vi "ShoulderNetwork.vi"(8 "error in (no error)":errorcluster) -> (0 "error out":errorcluster)   [LabVIEW 2023]
uses:
  Elevator/ElevatorGlobal.vi
  <vilib>/Rock Robotics/Network Tables/NT Write Boolean.vi
  <vilib>/Rock Robotics/Network Tables/NT Write Number.vi
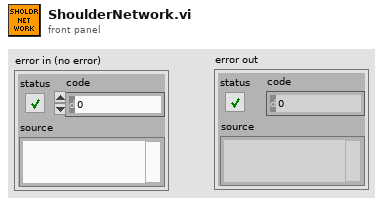
[diagram p1: front panel]
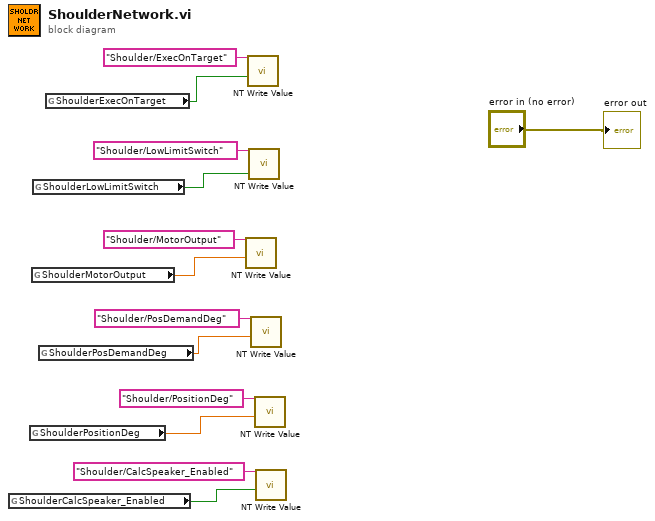
[diagram p0: block diagram]
diagram:
  n1 = global read "ElevatorGlobal.vi" "ShoulderCalcSpeaker_Enabled"() -> (w9:bool)
  n2 = global read "ElevatorGlobal.vi" "ShoulderPositionDeg"() -> (w5:dbl)
  n3 = global read "ElevatorGlobal.vi" "ShoulderMotorOutput"() -> (w3:dbl)
  n4 = global read "ElevatorGlobal.vi" "ShoulderLowLimitSwitch"() -> (w2:bool)
  n5 = global read "ElevatorGlobal.vi" "ShoulderPosDemandDeg"() -> (w4:dbl)
  n6 = global read "ElevatorGlobal.vi" "ShoulderExecOnTarget"() -> (w1:bool)
  n7 = call-poly <vilib>:"NT Write Value.vi"("value"=w3, "name"="Shoulder/MotorOutput") -> ()  [unwired: 9 in, 1 out]
  n8 = call-poly <vilib>:"NT Write Value.vi"("value"=w1, "name"="Shoulder/ExecOnTarget") -> ()  [unwired: 9 in, 1 out]
  n9 = call-poly <vilib>:"NT Write Value.vi"("value"=w2, "name"="Shoulder/LowLimitSwitch") -> ()  [unwired: 9 in, 1 out]
  n10 = call-poly <vilib>:"NT Write Value.vi"("value"=w4, "name"="Shoulder/PosDemandDeg") -> ()  [unwired: 9 in, 1 out]
  n11 = call-poly <vilib>:"NT Write Value.vi"("value"=w5, "name"="Shoulder/PositionDeg") -> ()  [unwired: 9 in, 1 out]
  n12 = call-poly <vilib>:"NT Write Value.vi"("value"=w9, "name"="Shoulder/CalcSpeaker_Enabled") -> ()  [unwired: 9 in, 1 out]
  "error out" <- "error in (no error)"
